vi "Read manipulator Operation.vi"(8 "Command Info":T5) -> (0 "Command Info":T5, 1 "SubSystem Data":T1={"Operation"=enum."Reserve", "Immediate Parameters"={"Wrist Power"=0.0, "Cascade Power"=0.0}, "Griddy Parameters"={"Griddy Command"=enum."idle", "Flip Wrist?"=FALSE}, "Reset Parameters"={"Reset Wrist"=FALSE, "Reset Cascade"=FALSE}, "Shoot Cube Parameters"={"Shot Preset"=enum."shoot mid"}}, 2 "Command Timing":cluster{"Start Time (ms)":u32, "Iterations":i32})   [LabVIEW 2020]
doc: "This returns the most recently scheduled command. This doesn't indicate whether the command finished and is running the default command."
uses:
  <vilib>/Rock Robotics/WPI/Framework/Command Status Info.ctl
  <vilib>/Rock Robotics/WPI/Framework/Completion Status.ctl
  <vilib>/Rock Robotics/WPI/Framework/Completion Notifier.ctl
  Implementation/manipulator Setpoints.ctl
  Implementation/manipulator Operations.ctl
  Implementation/Typedefs/Teleop Manipulator Commands.ctl
  Implementation/Typedefs/Cube Shooting Presets.ctl
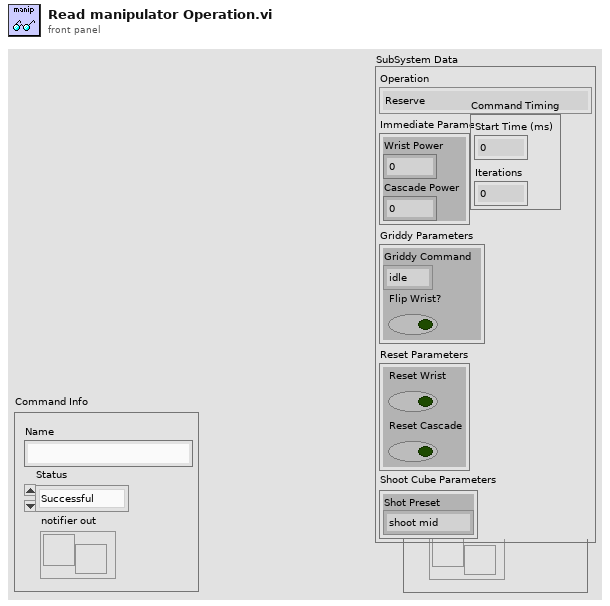
[diagram p1: front panel]
types:
  T1 = typedef "manipulator Setpoints.ctl" = cluster{"Operation":T2, "Immediate Parameters":cluster{"Wrist Power":dbl, "Cascade Power":dbl}, "Griddy Parameters":cluster{"Griddy Command":T3, "Flip Wrist?":bool}, "Reset Parameters":cluster{"Reset Wrist":bool, "Reset Cascade":bool}, "Shoot Cube Parameters":cluster{"Shot Preset":T4}}
  T2 = typedef "manipulator Operations.ctl" = enum16{"Reserve", "Read Current", "Immediate", "Reset Manipulator", "Grid-dy", "Shoot Cubes"}
  T3 = typedef "Teleop Manipulator Commands.ctl" = enum16{"idle", "intake cone sideways", "intake cone upright", "intake cone feeder", "intake cube feeder", "intake cube", "score low cone", "score low cube", "score mid cone", "score mid cube", "score high cone", "score high cube", "score mid cone up"}
  T4 = typedef "Cube Shooting Presets.ctl" = enum16{"shoot low", "shoot mid", "shoot high"}
  T5 = typedef "Command Status Info.ctl" = cluster{"Name":string, "Status":T6, "notifier out":T7}
  T6 = typedef "Completion Status.ctl" = enum16{"Successful", "Aborted", "Incomplete"}
  T7 = typedef "Completion Notifier.ctl" = refnum<notifier>
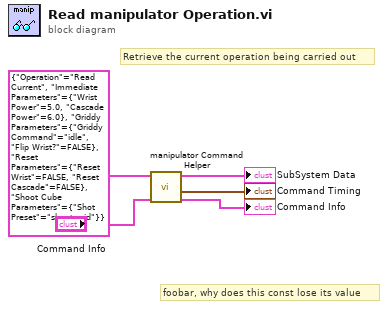
[diagram p0: block diagram]
diagram:
  # "foobar, why does this const lose its value"
  # "Retrieve the current operation being carried out"
  n1 = call "manipulator Command Helper.vi"("Command Info In"="Command Info", "SubSystem Data"=T1 {"Operation"=enum."Read Current", "Immediate Parameters"={"Wrist Power"=5.0, "Cascade Power"=6.0}, "Griddy Parameters"={"Griddy Command"=enum."idle", "Flip Wrist?"=FALSE}, "Reset Parameters"={"Reset Wrist"=FALSE, "Reset Cascade"=FALSE}, "Shoot Cube Parameters"={"Shot Preset"=enum."shoot mid"}}) -> ("Command Info Out"=→"Command Info":T5, "Command Timing"=→"Command Timing":cluster{"Start Time (ms)":u32, "Iterations":i32}, "SubSystem Data"=→"SubSystem Data":T1)  [unwired: 7 in]
